vi "Cylinder Trigger.vi"(7 "settings.<user name>":T5, 8 "register bus":T3={"Speed"="Speed", "Crank Angle"="Crank Angle", "Cycle Angle"="Cycle Angle", "Crank Count"="Crank Count", "Cycle Count"="Cycle Count", "1.25 MHz Counter"="625 kHz Counter", "Crank Rollover"="Crank Rollover", "Cycle Rollover"="Cycle Rollover", "shared settings"={"start"=0.0, "stuck limit"=0.0}} {"shared settings"."start" format="%#.15g"}, 11 "input.<user name>":T1={"probability compare"=65535, "high freq scaler"=0.0, "trigger position"=0}) -> (3 "triggered knock data":T2)   [LabVIEW 2013, in "Engine Simulation Toolkit.lvlib" / "Knock Sensor.lvlib"]
doc: "Determines if a high frequency knock component should be triggered for a given cylinder.\n\n<b>settings.<user name></b> - settings for the component. NI VeriStand will set these values. Create a control for this input. Replace <user name> with the name you wish this component to display as inside NI VeriStand. Make this name consistent for all controls, indicators, for all VIs of this component.\n<b>input.<user name></b> - input for the component. NI VeriStand will set these values. Create a control for this input. Replace <user name> with the name you wish this component to display as inside NI VeriStand. Make this name consistent for all controls, indicators, for all VIs of this component.\n<b>register bus</b> - connect this input to the output of the initialize APU VI. This contains references to APU state variables like position and speed.\n\n<b>triggered knock data</b> - data about the cylinder's knock status sent to the Generate Signal.vi"
uses:
  Knock Sensor.lvlib
  Cylinder Settings.ctl
  APU/Register Bus.ctl
  APU/Shared Settings.ctl
  Triggered Cylinder Data.ctl
  Cylinder Input.ctl
  <vilib>/Platform/TimedLoop/XDataNode/timing_clust.ctl
  <vilib>/Platform/TimedLoop/XDataNode/nitl_modes.ctl
  <vilib>/Platform/TimedLoop/XDataNode/wakeup.ctl
  <vilib>/rvi/Emulation/niFpgaSctlEmulationGetInTimedLoop.vi
  <vilib>/rvi/Emulation/niFpgaEmulationReportErrorSimple.vi
  <vilib>/rvi/Emulation/niFpgaGetClockAttributes.vi
  <vilib>/rvi/Emulation/niFpgaCriticalErrorInLSC.vi
  <vilib>/rvi/DataTransferAndStorage/Container/Common/niFpgaContainerExecOnDevCompGetState.vi
  <vilib>/rvi/DataTransferAndStorage/Register/Emulation/niFpgaRegisterEmulationFpgaImpl.vi
  <instcachedir>/0/niFpgaRegisterEmulationFpgaImpl_DCF4BC0110594B98B44A971D60CEEC4D.lvgen/niFpgaRegisterEmulationFpgaImpl_DCF4BC0110594B98B44A971D60CEEC4D_006.vi
  <vilib>/rvi/DataTransferAndStorage/Container/Common/niFpgaContainerGetUniqueNameForEmu.vi
  <vilib>/Platform/TimedLoop/XDataNode/XDataNode.xnode
  <vilib>/rvi/DataTransferAndStorage/Container/XNode/niFpgaContainer.xnode
  <vilib>/rvi/DataTransferAndStorage/Register/Emulation/niFpgaRegisterEmulationRefIn.vi
  <vilib>/Platform/TimedLoop/XDataNode/XDNodeRunTimeDep.lvlib
  Engine Simulation Toolkit.lvlib
  APU/APU.lvlib
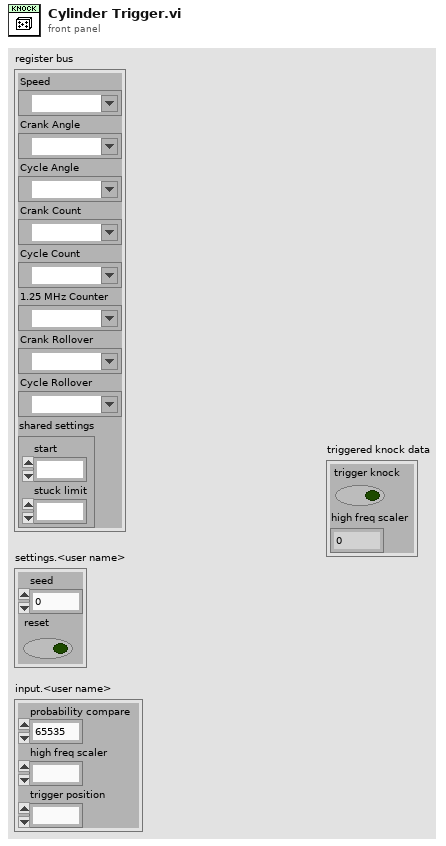
[diagram p1: front panel]
types:
  T1 = typedef "Engine Simulation Toolkit.lvlib/Knock Sensor.lvlib/Cylinder Input.ctl" = cluster{"probability compare":u16, "high freq scaler":fxp<+,10,0>, "trigger position":u16}
  T2 = typedef "Engine Simulation Toolkit.lvlib/Knock Sensor.lvlib/Triggered Cylinder Data.ctl" = cluster{"trigger knock":bool, "high freq scaler":fxp<+,10,0>}
  T3 = typedef "Engine Simulation Toolkit.lvlib/APU.lvlib/Register Bus.ctl" = cluster{"Speed":refnum<k21>, "Crank Angle":refnum<k21>, "Cycle Angle":refnum<k21>, "Crank Count":refnum<k21>, "Cycle Count":refnum<k21>, "1.25 MHz Counter":refnum<k21>, "Crank Rollover":refnum<k21>, "Cycle Rollover":refnum<k21>, "shared settings":T4}
  T4 = typedef "Engine Simulation Toolkit.lvlib/APU.lvlib/Shared Settings.ctl" = cluster{"start":fxp<+,17,17>, "stuck limit":fxp<+,18,18>}
  T5 = typedef "Engine Simulation Toolkit.lvlib/Knock Sensor.lvlib/Cylinder Settings.ctl" = cluster{"seed":u16, "reset":bool}
  T6 = typedef "XDNodeRunTimeDep.lvlib/timing_clust.ctl" = cluster{"Expected End [f-1]":u64, "Actual End [f-1]":u64, "Finished Late? [f-1]":bool, "Expected End [i-1]":u64, "Actual End [i-1]":u64, "Finished Late? [i-1]":bool, "Expected Start [i]":u64, "Actual Start [i]":u64, "Expected Start [f]":u64, "Actual Start [f]":u64, "Source Name":string, "Structure Name":string, "Period":i64, "Deadline":i64, "Offset":i64, "Start":i64, "Priority":i32, "Timeout":i32, "Mode":T7, "Wakeup Reason":T8, "Error":errorcluster, "Source Type":string, "Secondary Source Type":string, "Global End Time":u64, "Global Start Time":u64, "Frame Duration":u64, "Iteration Duration":u64, "Assigned CPU":i32, "I/O Scan Engine Mode":u32}
  T7 = typedef "XDNodeRunTimeDep.lvlib/nitl_modes.ctl" = enum32{"No Change", "Process missed periods, maintain original phase", "Discard missed periods, maintain original phase", "Process missed periods, ignore original phase", "Discard missed periods, ignore original phase"}
  T8 = typedef "XDNodeRunTimeDep.lvlib/wakeup.ctl" = enum32{"Normal", "Aborted", "Asynchronous wakeup", "Timing source error", "Timed loop error", "Timeout"}
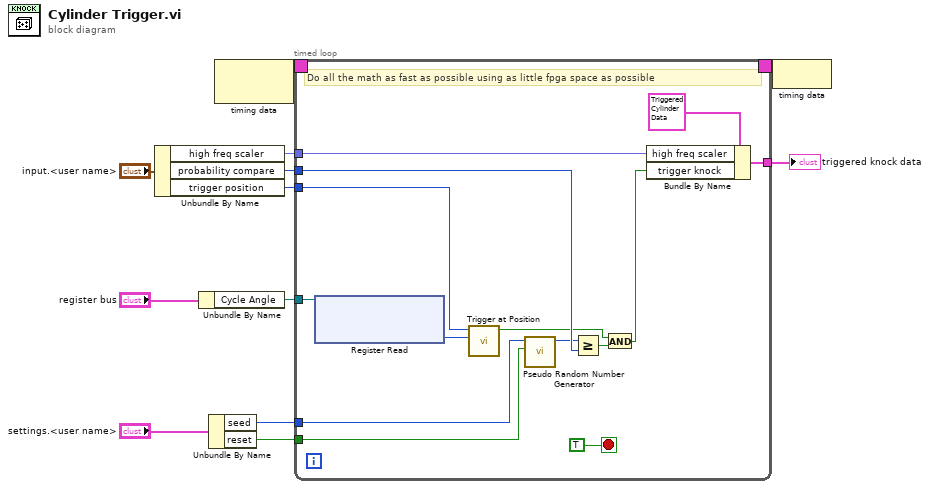
[diagram p0: block diagram]
diagram:
  n1 = Unbundle By Name("input.<user name>") -> ("high freq scaler"=w6:fxp<+,10,0>, "probability compare"=w5:u16, "trigger position"=w2:u16)
  n2 = Unbundle By Name("register bus") -> ("Cycle Angle"=w11:refnum<k21>)
  n3 = Unbundle By Name("settings.<user name>") -> ("seed"=w10:u16, "reset"=w1:bool)
  n4 = node-c288() -> (w4:T6)  [unwired: 1 in]
  n5 = timed-loop {
    timing: w4 -> [_]
    timing-out: [_] -> w3
    tunnel: w11 -> [w26]
    tunnel: w10 -> [w15]
    tunnel: [w24] -> w9
    tunnel: w6 -> [w21]
    tunnel: w5 -> [w20]
    tunnel: w2 -> [w16]
    tunnel: w1 -> [w13]
    stop <- TRUE stop-if-true
    # "Do all the math as fast as possible using as little fpga space as possible"
    n6 = xnode ("Register Read")("Register In"=w26) -> ("Data"=w22:u16)  [unwired: 1 out]
    n7 = call "Trigger at Position.vi"("position"=w22, "trigger position"=w16) -> ("trigger"=w17:bool)  [unwired: 9 in]
    n8 = call "Pseudo Random Number Generator.vi"("reset"=w13, "seed"=w15) -> ("pseudo random value"=w14:u16)  [unwired: 9 in]
    n9 = Greater Or Equal?(x=w14, y=w20) -> (x >= y?=w23:bool)
    n10 = And(x=w17, y=w23) -> (x .and. y?=w18:bool)
    n11 = Bundle By Name(cluster=T2 {"trigger knock"=FALSE, "high freq scaler"=0.0} ("Cylinder Knock State"), "high freq scaler"=w21, "trigger knock"=w18) -> (w24:T2)
  }
  "triggered knock data" <- w9
  n12 = node-c288(w3) -> ()
